vi "LVClass_CorrectionDataManager GetGreatestCommonPupil.vi"(0 "CorrectionDataManager in":refnum<class "CorrectionDataManager.lvclass">, 5 "Pupil in":refnum<class "Pupil.lvclass">, 11 "error in (no error)":errorcluster) -> (4 "CorrectionDataManager out":refnum<class "CorrectionDataManager.lvclass">, 6 "Pupil out":refnum<class "Pupil.lvclass">, 15 "error out":errorcluster)   [LabVIEW 2020, in "CorrectionDataManager.lvclass"]
doc: "Get the greatest common pupil from AOC data.\n\n<B>corrdata_managerIn</B> : CorrDataManager object.\n<B>corrdata_managerOut</B> : CorrDataManager object.\n<B>pupil in</B> : Pupil object to store the greatest common pupil\n<B>pupil out</B> : Pupil object has been upadtaed with the greatest common pupil"
uses:
  CorrectionDataManager.lvclass
  Pupil.lvclass
  CorrectionDataManager.lvclass/CorrectionDataManager.ctl
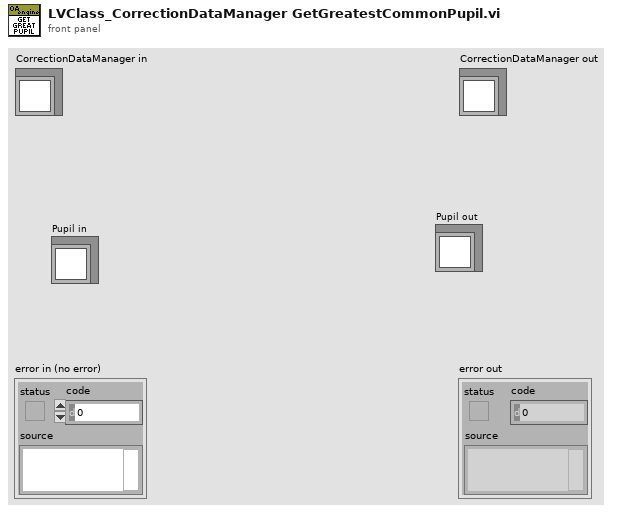
[diagram p1: front panel]
types:
  T1 = typedef "ClassID.ctl" = i64
  T2 = typedef "General dimensions definition.ctl" = cluster{"Size":T3, "Step":T4}
  T3 = typedef "Point2D.ctl" = cluster{"X":u32, "Y":u32}
  T4 = typedef "Point2Df.ctl" = cluster{"X":sgl, "Y":sgl}
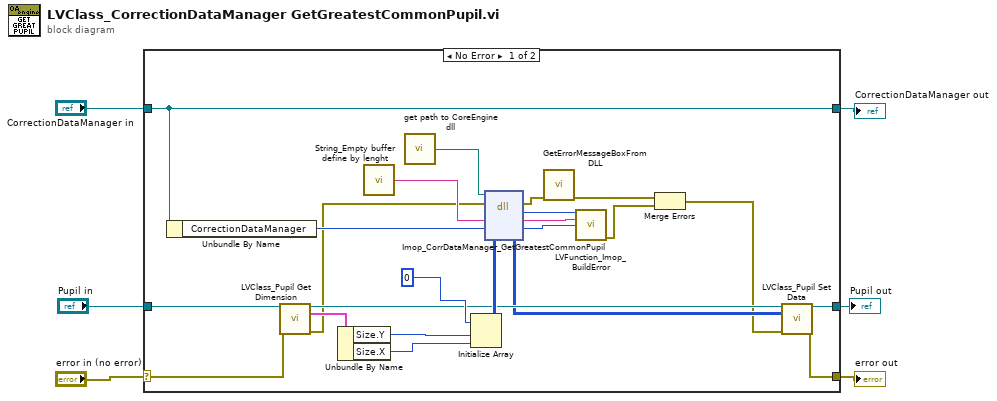
[diagram p0: block diagram]
diagram:
  n1 = case shown="No Error" "error in (no error)" {
    selector: "error in (no error)" -> [w11 w32]
    tunnel: [w8 w32] -> w4
    tunnel: [w22 w31] -> w5
    tunnel: "CorrectionDataManager in" -> [w22 w31]
    tunnel: "Pupil in" -> [w20 w30]
    tunnel: [w10 w30] -> w1
    frame No Error {
      n2 = Unbundle By Name(w22) -> ("CorrectionDataManager"=w21:T1)
      n3 = call "LVClass_Pupil Get Dimension.vi"("Pupil in"=w20, "error in (no error)"=w11) -> ("Pupil out"=w14:refnum<class "Pupil.lvclass">, "Dimension"=w19:T2, "error out"=w12:errorcluster)  [unwired: 11 in]
      n4 = Unbundle By Name(w19) -> ("Size.Y"=w17:u32, "Size.X"=w16:u32)
      n5 = call "String_Empty buffer define by lenght.vi"() -> ("Empty buffer"=w27:string)  [unwired: 1 in]
      n6 = call "get path to CoreEngine dll.vi"() -> ("path to wavekit library"=w23:path)  [unwired: 14 in, 1 out]
      n7 = Initialize Array(u8 0, w17, w16) -> (w15:u8[][])
      n8 = dll-call lib="D:/soft/HASO_v3/SVN_trunk/ImOpCoreEngine4_LV2011/DLLs/c_interface_vc100.dll" fn="Imop_CorrDataManager_GetGreatestCommonPupil"(path in=w23, error in=w12, "message"=w27, "corrdata_manager"=w21, "pupil"=w15) -> (error out=w26:errorcluster, "return type"=w29:i32, "message"=w28:string, "corrdata_manager"=w7:i64, "pupil"=w13:u8[][])  [unwired: 1 in, 1 out]
      n9 = call "GetErrorMessageBoxFromDLL.vi"("error IN"=w26) -> ("error OUT"=w25:errorcluster)  [unwired: 10 in]
      n10 = call "LVFunction_Imop_BuildError.vi"("code"=w29, "String to Prepend to source (\"\")"=w28, "Adresse"=w7) -> ("error out"=w24:errorcluster)  [unwired: 12 in]
      n11 = Merge Errors(w25, w24) -> (w9:errorcluster)
      n12 = call "LVClass_Pupil Set Data.vi"("Pupil in"=w14, "Data"=w13, "error in (no error)"=w9) -> ("Pupil out"=w10:refnum<class "Pupil.lvclass">, "error out"=w8:errorcluster)  [unwired: 11 in]
    }
    frame Error {
    }
  }
  "error out" <- w4
  "CorrectionDataManager out" <- w5
  "Pupil out" <- w1
